vi "GServer_Constructor.vi"(8 "error in (no error)":errorcluster, 11 "Gserver in":refnum<class "Gserver.lvclass">) -> (0 "error out":errorcluster, 3 "Gserver out":refnum<class "Gserver.lvclass">)   [LabVIEW 2014, in "Gserver.lvclass"]
doc: "Constructor of the Gserver class."
uses:
  Gserver.lvclass
  controls/Typedef_Gviewer-Query.ctl
  controls/Typedef_QueryType.ctl
  controls/Typedef_Gserver-init.ctl
  Gserver.lvclass/Gserver.ctl
  FAMM/FAMM.lvclass
  Common/controls/Global-services.vi
  Vsolver/Vsolver.lvclass
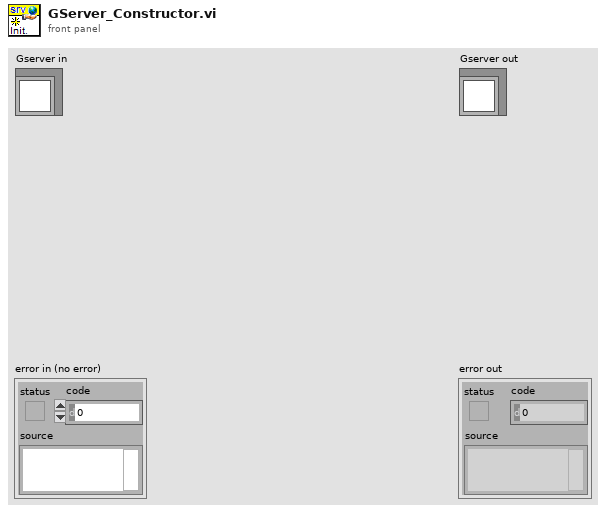
[diagram p1: front panel]
types:
  T1 = typedef "Typedef_Gserver-init.ctl" = enum16{"InitStarted", "FAMM_started", "HISW_Started", "Active"}
  T2 = typedef "Gserver.lvclass/Typedef_Gviewer-Query.ctl" = cluster{"Query_type":T3, "data":variant, "Source":string, "Time Stamp":timestamp}
  T3 = typedef "Gserver.lvclass/Typedef_QueryType.ctl" = enum16{"Subscribe", "DataRequest", "SetFAMMobject", "GetFAMMobject", "CloseClient", "Close Gserver"}
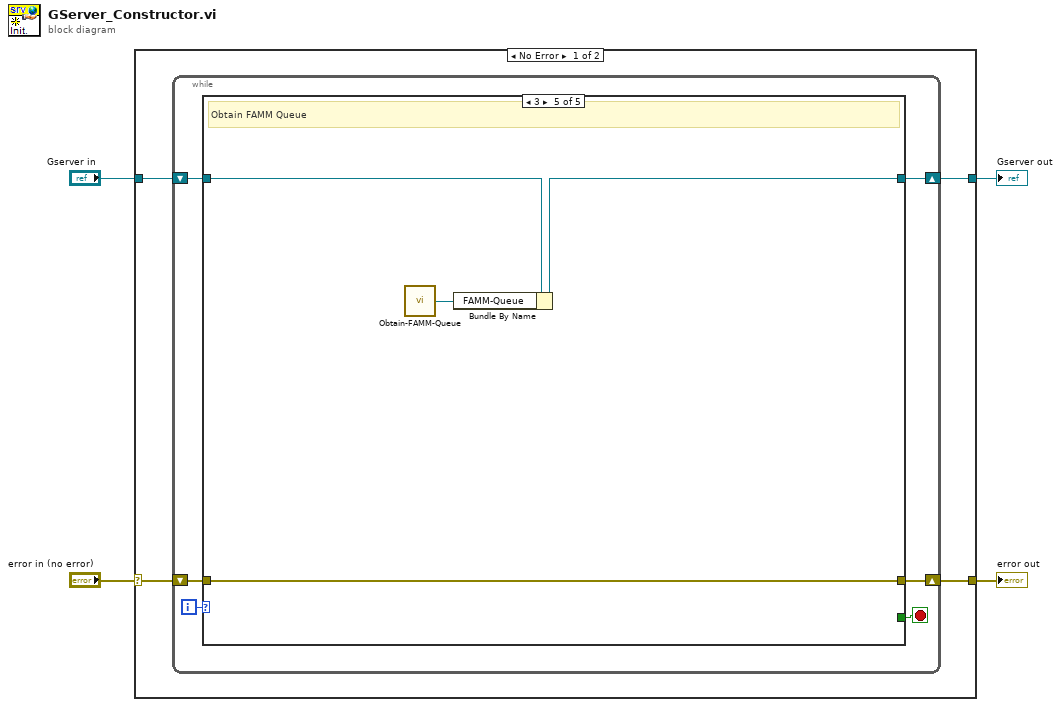
[diagram p0: block diagram]
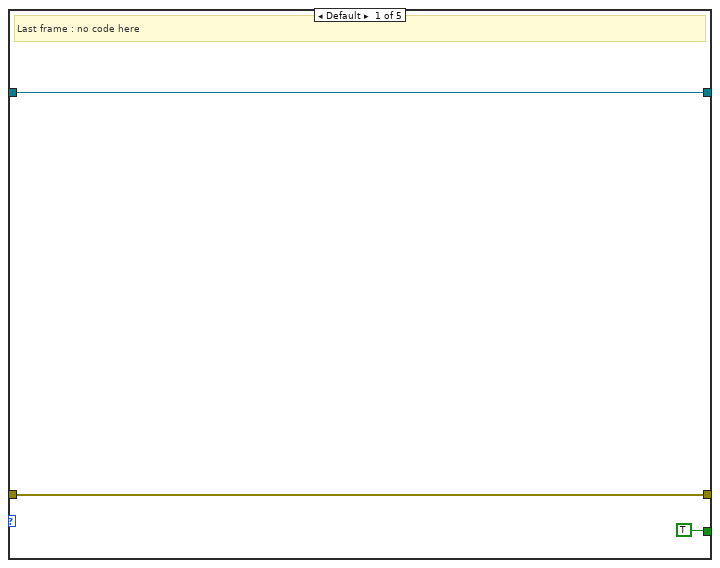
[diagram p2: hidden frame]
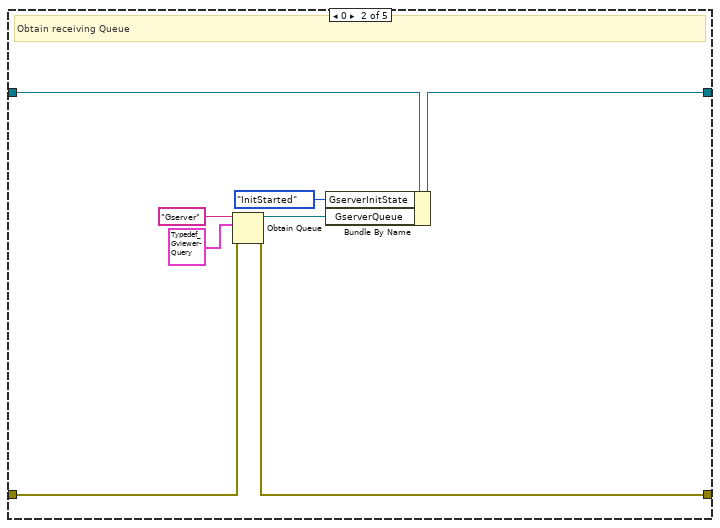
[diagram p3: hidden frame]
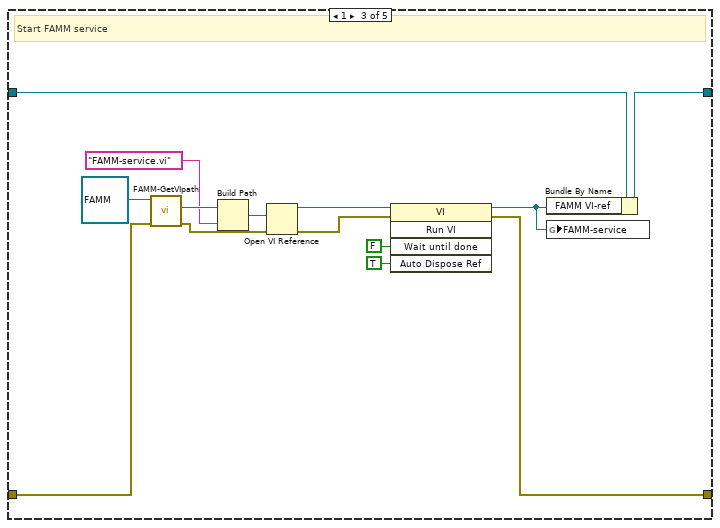
[diagram p4: hidden frame]
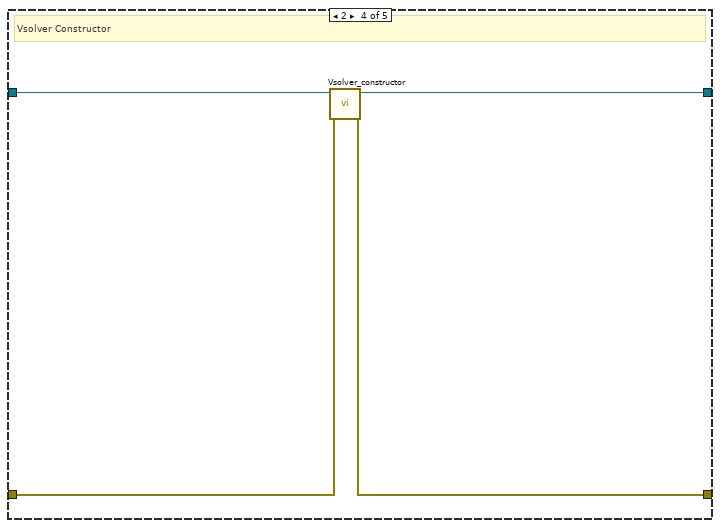
[diagram p5: hidden frame]
diagram:
  n1 = case shown="No Error" "error in (no error)" {
    selector: "error in (no error)" -> [w7 w49]
    tunnel: [w6 w49] -> w3
    tunnel: [w5 w48] -> w1
    tunnel: "Gserver in" -> [w8 w48]
    frame No Error {
      n2 = while {
        shift-right: [w9] -> w5
        shift-left: w8 -> [w10]
        shift-right: [w11] -> w6
        shift-left: w7 -> [w14]
        i -> [w13]
        stop <- w12 stop-if-true
        n3 = case shown="3" w13 {
          tunnel: w14 -> [w16 w23 w30 w43 w44]
          tunnel: [TRUE _ _ _ _] -> w12
          tunnel: [w16 w19 w29 w42 w44] -> w11
          tunnel: w10 -> [w15 w21 w28 w41 w47]
          tunnel: [w15 w20 w27 w40 w46] -> w9
          frame Default {
            # "Last frame : no code here"
          }
          frame 0 {
            # "Obtain receiving Queue"
            n4 = Obtain Queue(name (unnamed)="Gserver", element data type=T2 {"Query_type"=enum."DataRequest", "data"=variant, "Source"="", "Time Stamp"=timestamp(0 s since 1904-01-01)} ("Query"), error in (no error)=w23) -> (queue out=w22:refnum<queue>, error out=w19:errorcluster)  [unwired: 2 in, 1 out]
            n5 = Bundle By Name(cluster=w21, "GserverInitState"=Typedef_Gserver-init."InitStarted", "GserverQueue"=w22) -> (w20:refnum<class "Gserver.lvclass">)
          }
          frame 1 {
            # "Start FAMM service"
            n6 = call "FAMM-GetVIpath.vi"("error in (no error)"=w30, "FAMM in"=refnum<class "FAMM.lvclass"> refnum ("FAMM.lvclass")) -> ("error out"=w35:errorcluster, "MethodsPath"=w38:path)  [unwired: 7 in, 1 out]
            n7 = Build Path(base path=w38, name or relative path="FAMM-service.vi") -> (appended path=w36:path)
            n8 = Open VI Reference(vi path=w36, error in (no error)=w35) -> (vi reference=w34:refnum<vi>, error out=w33:errorcluster)  [unwired: 4 in]
            n9 = invoke class="VI" method="Run VI"(reference=w34, error in=w33, "Wait until done"=FALSE ("Wait Until Done"), "Auto Dispose Ref"=TRUE ("Auto Dispose Reference")) -> (reference out=w26:refnum<vi>, error out=w29:errorcluster)  [unwired: 1 in, 3 out]
            n10 = Bundle By Name(cluster=w28, "FAMM VI-ref"=w26) -> (w27:refnum<class "Gserver.lvclass">)
            n11 = global write "Global-services.vi" "FAMM-service"(w26) -> ()
          }
          frame 2 {
            # "Vsolver Constructor"
            n12 = call "Vsolver_constructor.vi"("error in (no error)"=w43, "Vsolver in"=w41) -> ("error out"=w42:errorcluster, "Vsolver out"=w40:refnum<class "Gserver.lvclass">)  [unwired: 8 in]
          }
          frame 3 {
            # "Obtain FAMM Queue"
            n13 = call "Obtain-FAMM-Queue.vi"() -> ("FAMM-Queue"=w45:refnum<queue>)  [unwired: 7 in]
            n14 = Bundle By Name(cluster=w47, "FAMM-Queue"=w45) -> (w46:refnum<class "Gserver.lvclass">)
          }
        }
      }
    }
    frame Error {
    }
  }
  "error out" <- w3
  "Gserver out" <- w1
